vi "replaceGoto.vi"(10 "String in":string) -> (2 "BotSpeak Out":string)   [LabVIEW 2014]
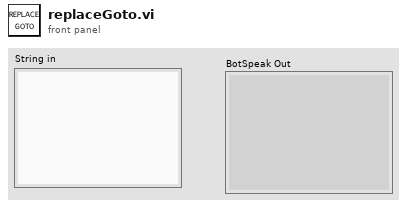
[diagram p1: front panel]
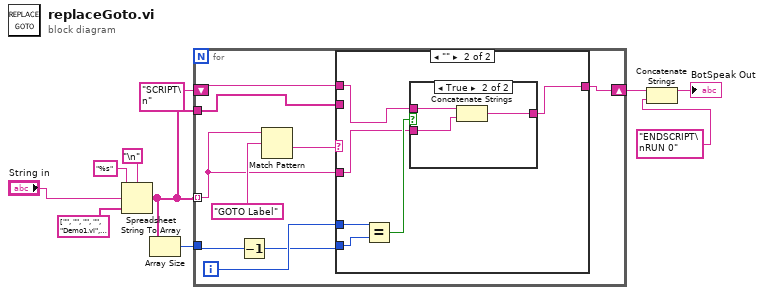
[diagram p0: block diagram]
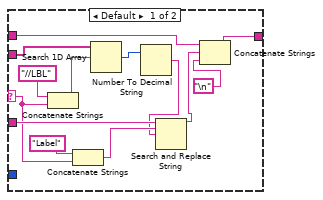
[diagram p2: hidden frame]
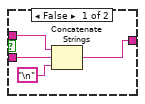
[diagram p3: hidden frame]
diagram:
  n1 = Spreadsheet String To Array(delimiter (Tab)="\n", format string="%s", spreadsheet string="String in", array type (2D Dbl)=string[] ["", "", "", "", "Demo1.vi", "DigitalWrite.vi", "VS_Wait.vi", ""] ("Array 3")) -> (array=w2:string[])
  n2 = Array Size(array=w2) -> (size(s)=w1:i32)
  n3 = for {
    tunnel: w2 -> [w15] mode=indexing
    tunnel: w2 -> [w19]
    shift-right: [w18] -> w5
    shift-left: "SCRIPT\n" -> [w17]
    tunnel: w1 -> [w11]
    i -> [w13]
    n4 = Decrement(x=w11) -> (x-1=w12:i32)
    n5 = Match Pattern(string=w15, regular expression="GOTO Label" ("search string/char (-)")) -> (after substring=w14:string)  [unwired: 1 in, 3 out]
    n6 = case shown="\"\"" w14 {
      selector: w14 -> [w28 _]
      tunnel: w19 -> [w32 _]
      tunnel: w15 -> [w29 w34]
      tunnel: [w21 w33] -> w18
      tunnel: w17 -> [w23 w35]
      tunnel: w13 -> [_ w38]
      tunnel: w12 -> [_ w37]
      frame Default {
        n7 = Concatenate Strings("//LBL" ("string"), w28) -> (w30:string)
        n8 = Concatenate Strings("Label" ("string"), w28) -> (w26:string)
        n9 = Search 1D Array(1D array=w32, element=w30) -> (index of element=w25:i32)  [unwired: 1 in]
        n10 = Number To Decimal String(number=w25) -> (decimal integer string=w24:string)  [unwired: 1 in]
        n11 = Search and Replace String(input string=w29, search string=w26, replace string=w24) -> (result string=w22:string)  [unwired: 5 in, 3 out]
        n12 = Concatenate Strings(w23, w22, "\n") -> (w21:string)
      }
      frame "" {
        n13 = Equal?(x=w38, y=w37) -> (x = y?=w36:bool)
        n14 = case shown="True" w36 {
          tunnel: w35 -> [w42 w45]
          tunnel: w34 -> [w41 w44]
          tunnel: [w39 w43] -> w33
          frame False {
            n15 = Concatenate Strings(w42, w41, "\n") -> (w39:string)
          }
          frame True {
            n16 = Concatenate Strings(w45, w44) -> (w43:string)
          }
        }
      }
    }
  }
  n17 = Concatenate Strings(w5, "ENDSCRIPT\nRUN 0" ("string")) -> (→"BotSpeak Out":string)
